vi "01 LinkTest.vi"(8 "error in (no error)":errorcluster caption="错误输入（无错误）", 9 "超时毫秒":i32, 10 "客服端参数":cluster{"本机端口":u16, "主机 IP":string, "主机端口":u16}={"本机端口"=0, "主机 IP"="0", "主机端口"=0}, 11 "TCPClientClass 输入":refnum<class "TCPClientClass.lvclass">) -> (0 "error out":errorcluster caption="错误输出", 2 "成功？":bool, 3 "TCPClientClass 输出":refnum<class "TCPClientClass.lvclass">)   [LabVIEW 2019, in "TCPClientClass.lvclass"]
uses:
  TCPClientClass.lvclass
  TCPClientClass.lvclass/TCPClientClass.ctl
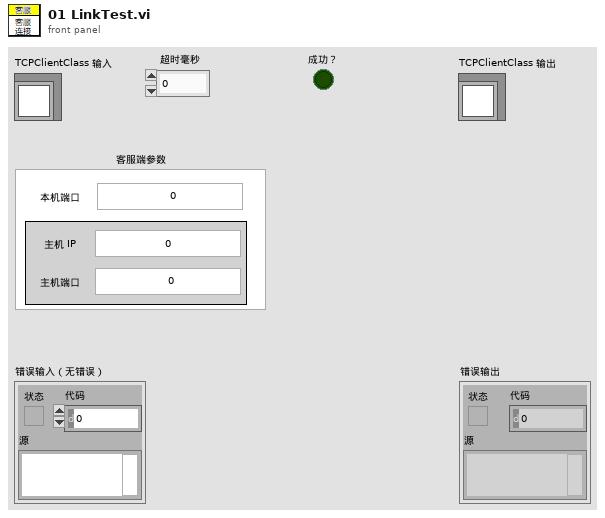
[diagram p1: front panel]
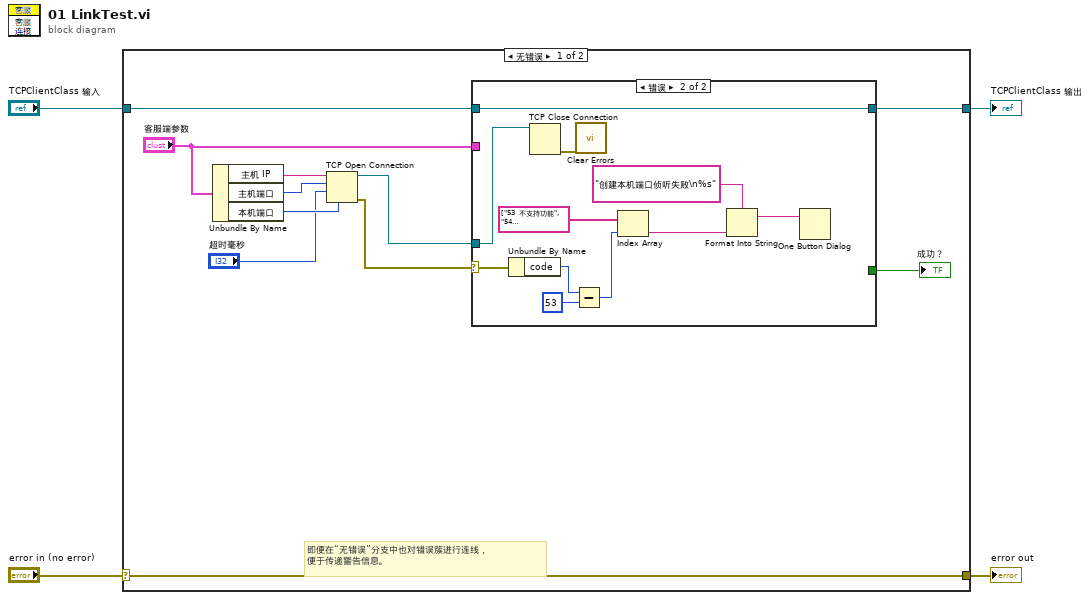
[diagram p0: block diagram]
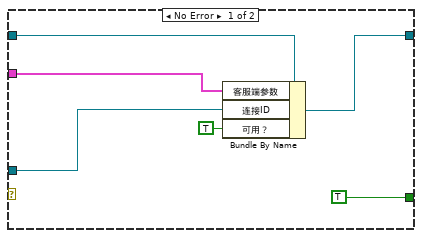
[diagram p2: hidden frame]
diagram:
  n1 = case shown="无错误" "error in (no error)" {
    selector: "error in (no error)" -> [w15 w34]
    tunnel: [w15 w34] -> w3
    tunnel: [w9 w33] -> w1
    tunnel: "TCPClientClass 输入" -> [w10 w33]
    frame No Error {
      # "即便在“无错误”分支中也对错误簇进行连线，\n便于传递警告信息。"
      n2 = Unbundle By Name("客服端参数") -> ("主机 IP"=w13:string, "主机端口"=w12:u16, "本机端口"=w14:u16)
      n3 = TCP Open Connection(address=w13, remote port or service name=w12, timeout ms (60000)="超时毫秒", local port=w14) -> (connection ID=w7:refnum<k5>, error out=w8:errorcluster)  [unwired: 1 in]
      n4 = case shown="错误" w8 {
        selector: w8 -> [_ w30]
        tunnel: w10 -> [w21 w24]
        tunnel: [w20 w24] -> w9
        tunnel: w7 -> [w19 w23]
        tunnel: [TRUE _] -> w5
        tunnel: "客服端参数" -> [w17 _]
        frame No Error {
          n5 = Bundle By Name(cluster=w21, "客服端参数"=w17, "连接ID"=w19, "可用？"=TRUE) -> (w20:refnum<class "TCPClientClass.lvclass">)
        }
        frame Error {
          n6 = Unbundle By Name(w30) -> ("code"=w32:i32)
          n7 = TCP Close Connection(connection ID=w23) -> (error out=w22:errorcluster)  [unwired: 2 in, 1 out]
          n8 = Subtract(x=w32, y=53) -> (x-y=w28:i32)
          n9 = call <vilib>:"Clear Errors.vi"("error in (no error)"=w22) -> ()  [unwired: 5 in, 2 out]
          n10 = Index Array(array=string[] ["53  不支持功能", "54  网络地址不合法", "55  网络运行正在进行中", "56  网络操作超过用户指定或系统时限", "57  网络连接繁忙", "58  系统不支持网络功能", "59  网络已关闭、无法到达或已重置", "60  指定的网络地址目前正在使用中", "61  系统无法分配必要的内存", "62  系统导致网络连接丢失", "63  服务器拒绝网络连接", "64  网络连接尚未建立", "65  网络连接已经建立", "66  网络连接被同行关闭"], index=w28) -> (element=w26:string)
          n11 = Format Into String(format string="创建本机端口侦听失败\n%s" ("格式字符串"), w26) -> (resulting string=w25:string)  [unwired: 2 in, 1 out]
          n12 = One Button Dialog(message=w25) -> ()  [unwired: 1 in, 1 out]
        }
      }
      "成功？" <- w5
    }
    frame Error {
    }
  }
  "error out" <- w3
  "TCPClientClass 输出" <- w1
